vi "CheckIfGoop2VI.vi"(1 "ViPath":path, 5 "error in (no error)":errorcluster) -> (15 "GOOP2Class":bool, 16 "ClassName":string, 17 "ClassPath":path, 19 "error out":errorcluster)   [LabVIEW 2020, in "ClassReader.lvclass"]
uses:
  ClassReader.lvclass
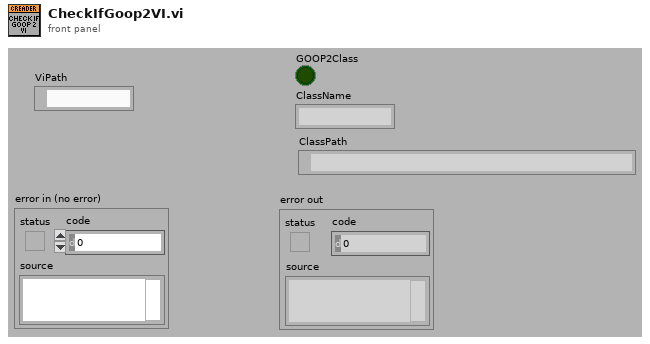
[diagram p1: front panel]
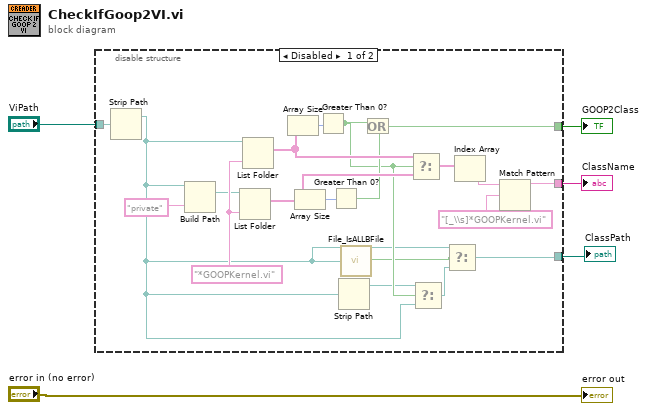
[diagram p0: block diagram]
diagram:
  n1 = disable-structure shown="Disabled" {
    disable-tunnel: [w14 _] -> w5
    disable-tunnel: [w13 _] -> w4
    disable-tunnel: "ViPath" -> [w12 _]
    disable-tunnel: [w6 _] -> w1
    frame Disabled {
      w23 = "*GOOPKernel.vi" ("pattern")
      n2 = Strip Path(path=w12) -> (stripped path=w8:path)  [unwired: 1 out]
      n3 = Build Path(base path=w8, name or relative path="private" ("element")) -> (appended path=w22:path)
      n4 = List Folder(path=w22, pattern=w23) -> (filenames=w20:string[])  [unwired: 2 in, 3 out]
      n5 = List Folder(path=w8, pattern=w23) -> (filenames=w19:string[])  [unwired: 2 in, 3 out]
      n6 = Array Size(array=w19) -> (size(s)=w21:i32)
      n7 = Array Size(array=w20) -> (size(s)=w24:i32)
      n8 = Greater Than 0?(x=w21) -> (x > 0?=w11:bool)
      n9 = Greater Than 0?(x=w24) -> (x > 0?=w18:bool)
      n10 = Strip Path(path=w8) -> (stripped path=w10:path)  [unwired: 1 out]
      n11 = call "File_IsALLBFile.vi"("path"=w8) -> ("path to VI library?"=w9:bool)
      n12 = Or(x=w11, y=w18) -> (x .or. y?=w14:bool)
      n13 = Select(t=w19, s=w11, f=w20) -> (s? t:f=w15:string[])
      n14 = Select(t=w10, s=w11, f=w8) -> (s? t:f=w7:path)
      n15 = Select(t=w8, s=w9, f=w7) -> (s? t:f=w6:path)
      n16 = Index Array(array=w15) -> (element=w17:string)  [unwired: 1 in]
      n17 = Match Pattern(string=w17, regular expression="[_\\s]*GOOPKernel.vi" ("pattern")) -> (before substring=w13:string)  [unwired: 1 in, 3 out]
    }
    frame Enabled {
    }
  }
  "GOOP2Class" <- w5
  "ClassName" <- w4
  "ClassPath" <- w1
  "error out" <- "error in (no error)"
